vi "FSM lab2.vi"() -> ()   [LabVIEW 2019]
uses:
  Control 1.ctl
panel:
  out "Humidity state":dbl
  out "Temp state":dbl
  out "State no":dbl
  out "Plant state":string
  in  "Moisture sensor":dbl(slide) scale=0.0..100.0 scale format="%#_3f"
  in  "Thermometer":dbl(slide) scale=-10.0..50.0 scale format="%#_3g"
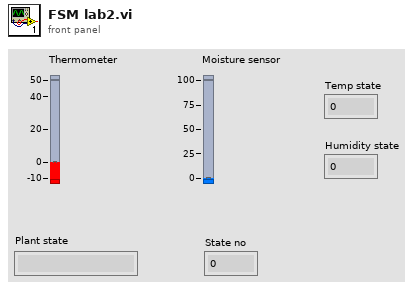
[diagram p1: front panel]
types:
  T1 = enum16{"SadPlant", "OkPlant", "HappyPlant", "AquireSensorData", "Init"}
  T2 = typedef "Control 1.ctl" = enum16{"Bad", "Ok", "Good"}
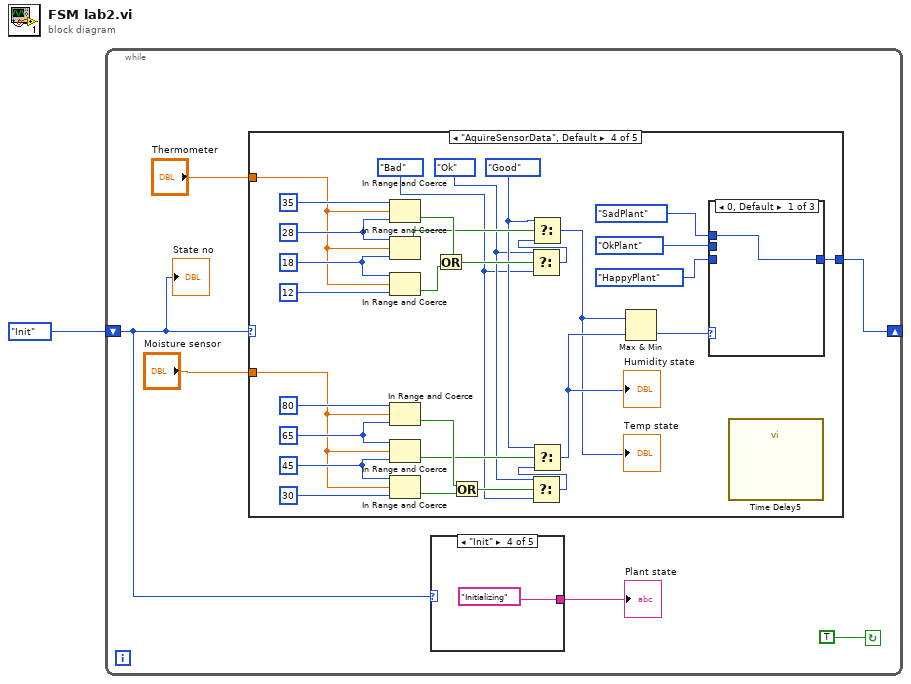
[diagram p0: block diagram]
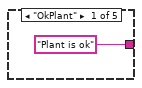
[diagram p2: hidden frame]
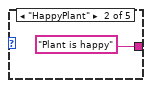
[diagram p3: hidden frame]
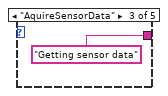
[diagram p4: hidden frame]
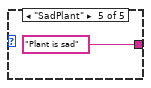
[diagram p5: hidden frame]
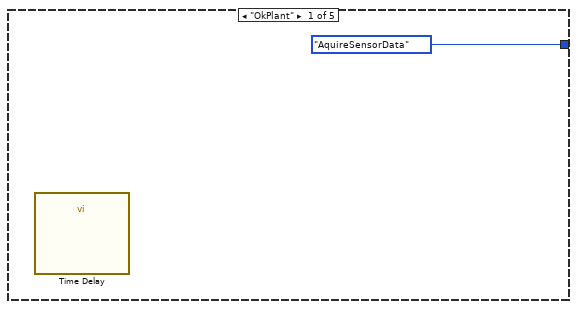
[diagram p6: hidden frame]
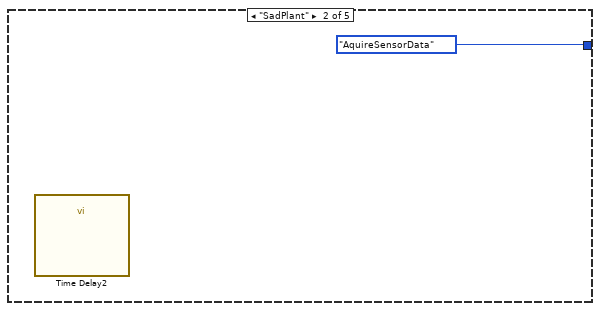
[diagram p7: hidden frame]
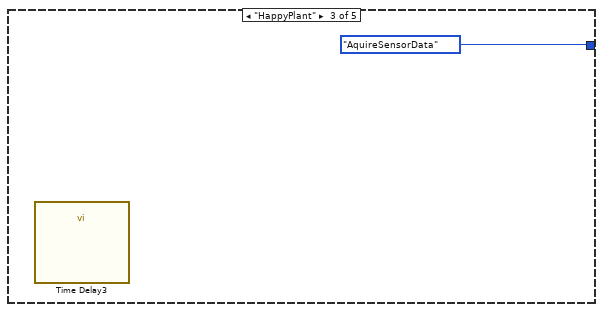
[diagram p8: hidden frame]
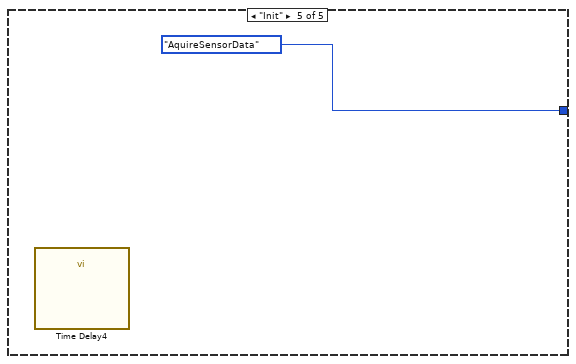
[diagram p11: hidden frame]
diagram:
  n1 = while {
    shift-right: [w7] -> _
    shift-left: T1."Init" -> [w2]
    stop <- TRUE continue-if-true
    n2 = case shown="\"AquireSensorData\", Default" w2 {
      tunnel: [T1."AquireSensorData" ("Enum") T1."AquireSensorData" ("Enum") T1."AquireSensorData" ("Enum") w34 T1."AquireSensorData" ("Enum")] -> w7
      tunnel: "Moisture sensor" -> [_ _ _ w41 _]
      tunnel: "Thermometer" -> [_ _ _ w22 _]
      frame "OkPlant" {
        n3 = call "Time Delay"() -> ()  [unwired: 11 in, 1 out]
      }
      frame "SadPlant" {
        n4 = call "Time Delay2"() -> ()  [unwired: 11 in, 1 out]
      }
      frame "HappyPlant" {
        n5 = call "Time Delay3"() -> ()  [unwired: 11 in, 1 out]
      }
      frame "AquireSensorData", Default {
        w27 = 18
        w28 = 28
        w18 = Control_1."Bad"
        w19 = Control_1."Ok"
        w20 = Control_1."Good"
        w42 = 45
        w43 = 65
        n6 = In Range and Coerce(upper limit=35, x=w22, lower limit=w28) -> (In Range?=w26:bool)  [unwired: 1 out]
        n7 = In Range and Coerce(upper limit=w28, x=w22, lower limit=w27) -> (In Range?=w24:bool)  [unwired: 1 out]
        n8 = In Range and Coerce(upper limit=w27, x=w22, lower limit=12) -> (In Range?=w25:bool)  [unwired: 1 out]
        n9 = In Range and Coerce(upper limit=80, x=w41, lower limit=w43) -> (In Range?=w40:bool)  [unwired: 1 out]
        n10 = In Range and Coerce(upper limit=w43, x=w41, lower limit=w42) -> (In Range?=w37:bool)  [unwired: 1 out]
        n11 = In Range and Coerce(upper limit=w42, x=w41, lower limit=30) -> (In Range?=w39:bool)  [unwired: 1 out]
        n12 = Or(x=w26, y=w25) -> (x .or. y?=w21:bool)
        n13 = Or(x=w40, y=w39) -> (x .or. y?=w38:bool)
        n14 = Select(t=w19, s=w21, f=w18) -> (s? t:f=w23:T2)
        n15 = Select(t=w19, s=w38, f=w18) -> (s? t:f=w36:T2)
        n16 = Select(t=w20, s=w24, f=w23) -> (s? t:f=w16:T2)
        "Temp state" <- w16
        n17 = Select(t=w20, s=w37, f=w36) -> (s? t:f=w17:T2)
        "Humidity state" <- w17
        n18 = Max & Min(x=w16, y=w17) -> (min(x,y)=w35:u16)  [unwired: 1 out]
        n19 = case shown="0, Default" w35 {
          tunnel: [w46 w47 w48] -> w34
          tunnel: T1."SadPlant" -> [w46 _ _]
          tunnel: T1."OkPlant" -> [_ w47 _]
          tunnel: T1."HappyPlant" -> [_ _ w48]
          frame 0, Default {
          }
          frame 1 {
          }
          frame 2 {
          }
        }
        n20 = call "Time Delay5"() -> ()  [unwired: 11 in, 1 out]
      }
      frame "Init" {
        n21 = call "Time Delay4"() -> ()  [unwired: 11 in, 1 out]
      }
    }
    n22 = case shown="\"Init\"" w2 {
      tunnel: ["Plant is ok" "Plant is happy" "Getting sensor data" "Initializing" "Plant is sad"] -> w3
      frame "OkPlant" {
      }
      frame "HappyPlant" {
      }
      frame "AquireSensorData" {
      }
      frame "Init" {
      }
      frame "SadPlant" {
      }
    }
    "Plant state" <- w3
    "State no" <- w2
  }
